vi "Shutdown.vi"(8 "error in":errorcluster, 11 "Manual UI in":refnum<class "Manual UI.lvclass">) -> (0 "error out":errorcluster, 3 "Manual UI out":refnum<class "Manual UI.lvclass">)   [LabVIEW 2019, in "Manual UI.lvlib" / "Manual UI.lvclass"]
doc: "Transmit a normal stop to all instantiated instrument Actors."
uses:
  Project/Manual UI.lvclass
  Project/Manual UI.lvclass/Manual UI.ctl
  builds/Engine/Actor Framework.lvlibp/1abvi3w/vi.lib/ActorFramework/Message Enqueuer/Message Enqueuer.lvclass
  builds/Engine/Actor Framework.lvlibp/1abvi3w/vi.lib/ActorFramework/Stop Msg/Stop Msg.lvclass
  builds/Engine/Engine.lvlibp/Project/Engine.lvclass
  C:/Users/Public/Documents/Development/builds/Engine/Engine.lvlibp/Project/Engine.lvclass
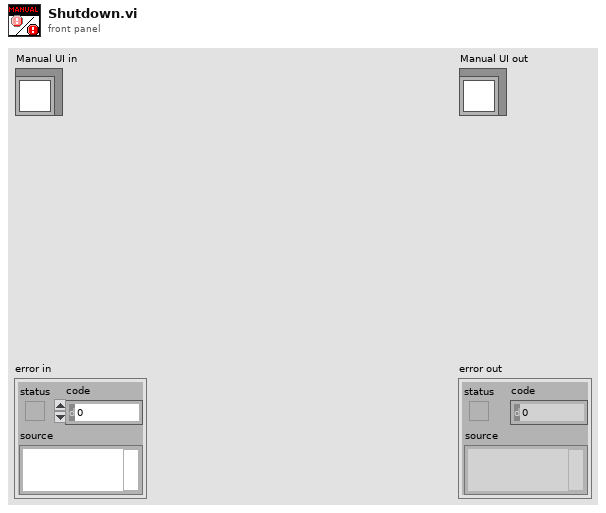
[diagram p1: front panel]
types:
  T1 = cluster{"Identifier":string, "Enqueuer":refnum<class "Message Enqueuer.lvclass">}[]
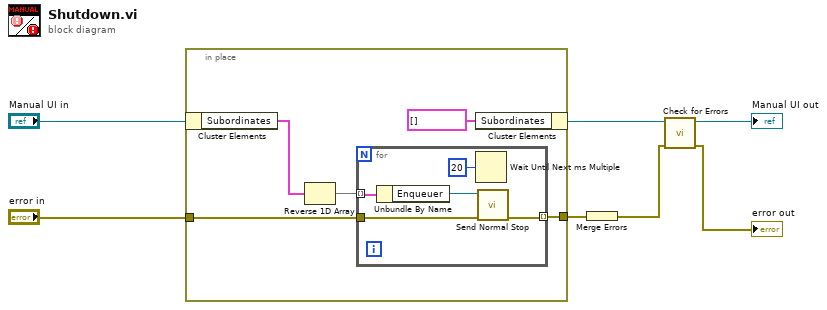
[diagram p0: block diagram]
diagram:
  n1 = in-place {
    in-place-border: "error in" -> [w10]
    in-place-border: [w9] -> w5
    n2 = in-place-cluster #1("Manual UI in") -> ("Subordinates"=w11:T1)
    n3 = Reverse 1D Array(array=w11) -> (reversed array=w8:T1)
    n4 = for {
      tunnel: w8 -> [w17] mode=indexing
      tunnel: w10 -> [w15]
      tunnel: [w14] -> w9 mode=indexing
      n5 = Unbundle By Name(w17) -> ("Enqueuer"=w16:refnum<class "Message Enqueuer.lvclass">)
      n6 = Wait Until Next ms Multiple(millisecond multiple=u32 20) -> ()  [unwired: 1 out]
      n7 = call "Send Normal Stop.vi"("error in (no error)"=w15, "Message Enqueuer"=w16) -> ("error out"=w14:errorcluster)  [unwired: 9 in]
    }
    n8 = in-place-cluster #1("Subordinates"=T1 []) -> (w4:refnum<class "Manual UI.lvclass">)
  }
  n9 = Merge Errors(w5) -> (w2:errorcluster)
  n10 = call "Check for Errors.vi"("error in"=w2, "Engine in"=w4) -> ("error out"=→"error out":errorcluster, "Engine out"=→"Manual UI out":refnum<class "Manual UI.lvclass">)  [unwired: 8 in]
